vi "APC_9049_SAVE_loop.vi"(0 "DAQqueues":T1) -> ()   [LabVIEW 2020]
doc: "This example demonstrates the procedure required to apply different NI-DAQmx Custom Scales to each virtual channel in a task. A DAQmx Task Property Node (Functions >> NI Measurements >> DAQmx - Data Acquisition >> DAQmx Advanced Task Options) is used to obtain the task's virtual channels. A DAQmx Channel Property Node (Functions >> NI Measurements >> DAQmx - Data Acquisition) is then used to set the custom scale for each virtual channel in the task.\n\nThe \"DAQmx Create Scale\" VI creates a custom scale for each channel in the channel list. *Note, make sure your Minimum and Maximum channel parameters are consistent with the range the scale will create."
uses:
  controls/APC_DAQqueues.ctl
  controls/APC_SavingFile.ctl
  <vilib>/Platform/TimedLoop/XDataNode/timing_clust.ctl
  <vilib>/Platform/TimedLoop/XDataNode/nitl_modes.ctl
  <vilib>/Platform/TimedLoop/XDataNode/wakeup.ctl
  <vilib>/platform/TimedLoop/XDataNode/XDataNode.xnode
  <vilib>/Platform/TimedLoop/XDataNode/XDNodeRunTimeDep.lvlib
panel:
  in  "BufferingTImeLimit [s]":i32
  out "SignalList.CycAvg":string[](array[string])
  out "Cycles to measure":u16
  out "# elements in queue":i32
  out "Recorded cycles":i32
  out "TEST CODE":string
  out "No disk":bool=TRUE
  out "Full disk":bool
  out "size(s) 2":i32[](array[numeric])
  out "size(s)":i32[](array[numeric])
  out "Files and paths":T2
  out "error out 2":errorcluster
  out "error out":errorcluster
  in  "PostMortem":bool
  in  "AutoClearNote":bool
  out "ID":u32=6
  out "Test Notes":string
  out "FLUSH and SAVE BUFFER":bool
  out "REC BUFFER":bool
  in  "Stop File Saving Loop":bool
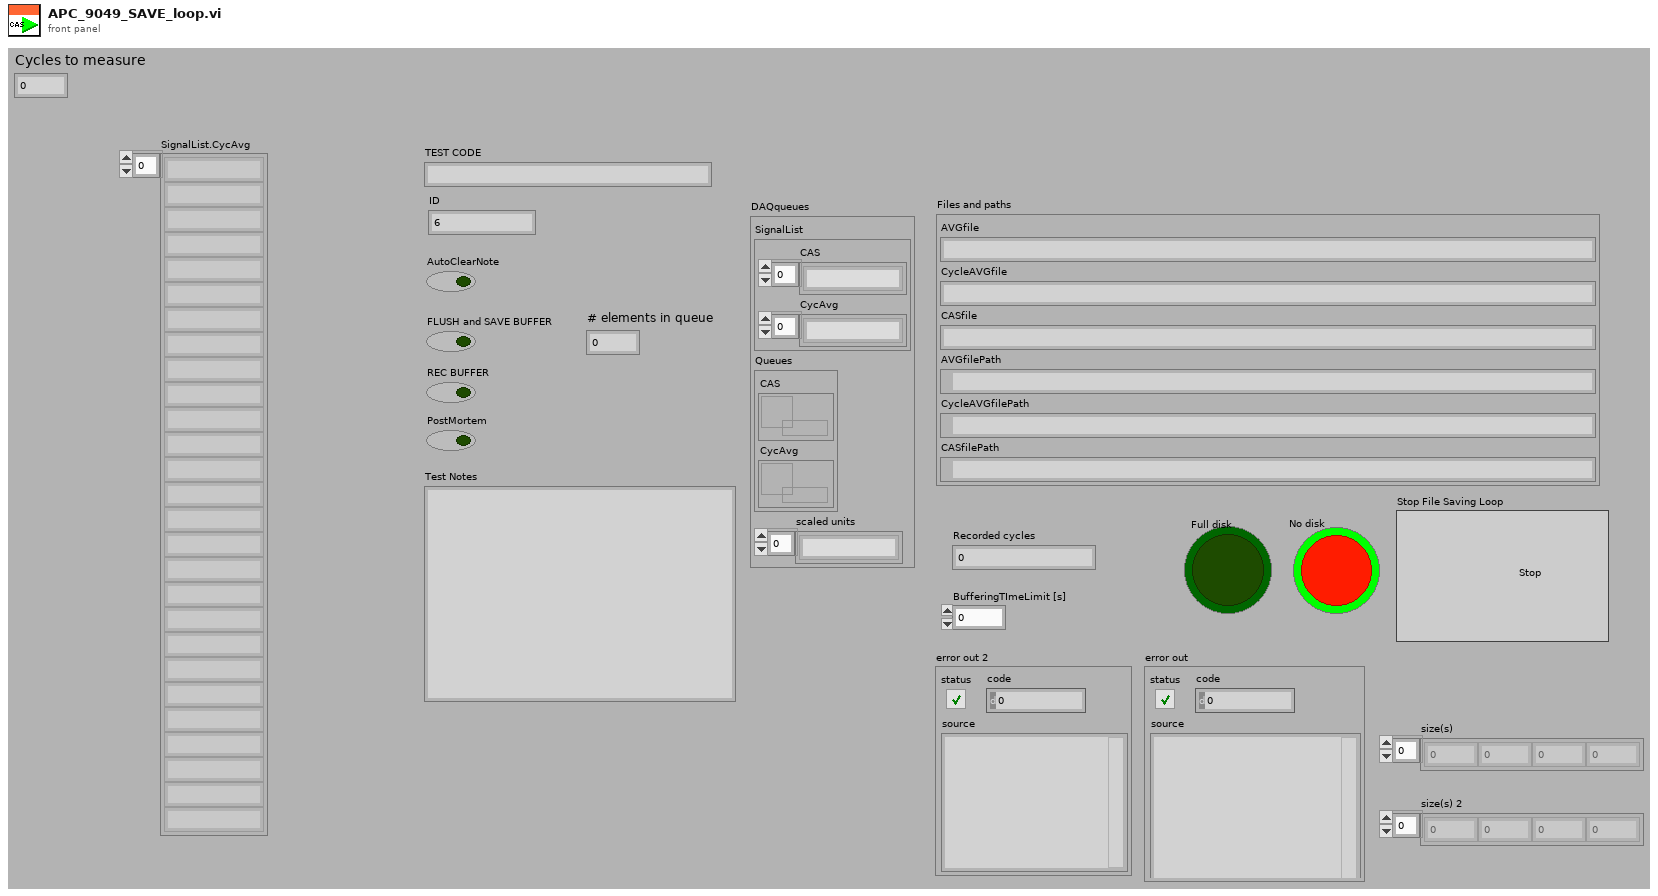
[diagram p1: front panel]
types:
  T1 = typedef "APC_DAQqueues.ctl" = cluster{"SignalList":cluster{"CAS":string[], "CycAvg":string[]}, "Queues":cluster{"CAS":refnum<queue>, "CycAvg":refnum<queue>}, "scaled units":string[]}
  T2 = cluster{"AVGfile":string, "CycleAVGfile":string, "CASfile":string, "AVGfilePath":path, "CycleAVGfilePath":path, "CASfilePath":path}
  T3 = enum16{"open", "open or create", "create or replace", "create", "open (read-only)"}
  T4 = typedef "XDNodeRunTimeDep.lvlib/timing_clust.ctl" = cluster{"Expected End [f-1]":u64, "Actual End [f-1]":u64, "Finished Late? [f-1]":bool, "Expected End [i-1]":u64, "Actual End [i-1]":u64, "Finished Late? [i-1]":bool, "Expected Start [i]":u64, "Actual Start [i]":u64, "Expected Start [f]":u64, "Actual Start [f]":u64, "Source Name":string, "Structure Name":string, "Period":i64, "Deadline":i64, "Offset":i64, "Start":i64, "Priority":i32, "Timeout":i32, "Mode":T5, "Wakeup Reason":T6, "Error":errorcluster, "Source Type":string, "Secondary Source Type":string, "Global End Time":u64, "Global Start Time":u64, "Frame Duration":u64, "Iteration Duration":u64, "Assigned CPU":i32, "I/O Scan Engine Mode":u32}
  T5 = typedef "XDNodeRunTimeDep.lvlib/nitl_modes.ctl" = enum32{"No Change", "Process missed periods, maintain original phase", "Discard missed periods, maintain original phase", "Process missed periods, ignore original phase", "Discard missed periods, ignore original phase"}
  T6 = typedef "XDNodeRunTimeDep.lvlib/wakeup.ctl" = enum32{"Normal", "Aborted", "Asynchronous wakeup", "Timing source error", "Timed loop error", "Timeout"}
  T7 = typedef "APC_SavingFile.ctl" = cluster{"TEST CODE":string, "ID":u32, "FLUSH and SAVE BUFFER":bool, "REC BUFFER":bool, "Test Notes":string, "Cycles":u16}
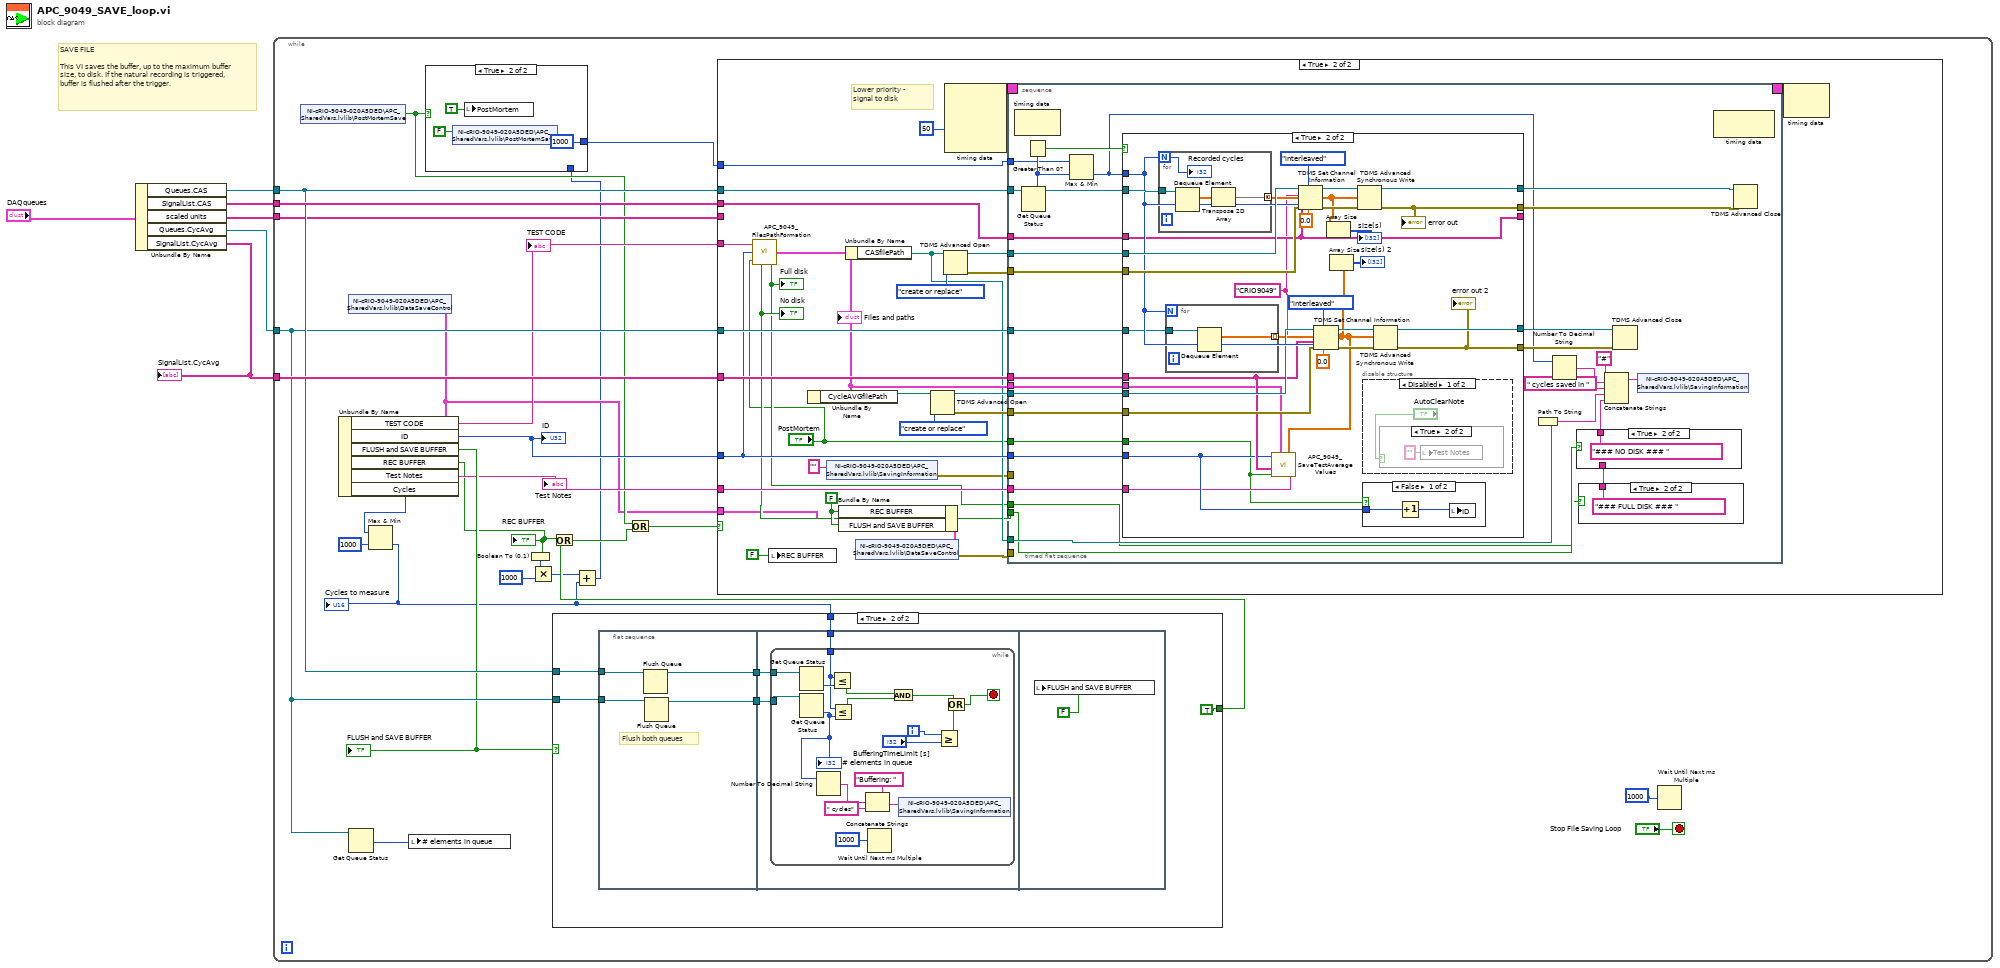
[diagram p0: block diagram]
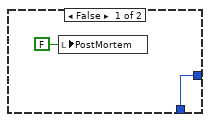
[diagram p2: hidden frame]
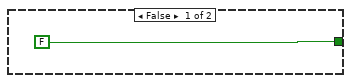
[diagram p3: hidden frame]
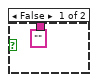
[diagram p5: hidden frame]
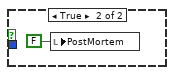
[diagram p10: hidden frame]
diagram:
  # "SAVE FILE\n\nThis VI saves the buffer, up to the maximum buffer size, to disk. If the natural recording is triggered, buffer is flushed after the trigger."
  n1 = Unbundle By Name("DAQqueues") -> ("Queues.CAS"=w6:refnum<queue>, "SignalList.CAS"=w5:string[], "scaled units"=w2:string[], "Queues.CycAvg"=w4:refnum<queue>, "SignalList.CycAvg"=w3:string[])
  "SignalList.CycAvg" <- w3
  n2 = while {
    tunnel: w6 -> [w28]
    tunnel: w5 -> [w32]
    tunnel: w4 -> [w25]
    tunnel: w3 -> [w30]
    tunnel: w2 -> [w26]
    stop <- "Stop File Saving Loop" stop-if-true
    n3 = shared-variable "NI-cRIO-9049-020A5DED\\APC_SharedVars.lvlib\\PostMortemSave"() -> (w12:bool)  [unwired: 1 in, 1 out]
    n4 = shared-variable "NI-cRIO-9049-020A5DED\\APC_SharedVars.lvlib\\DataSaveControl"() -> (w9:T7)  [unwired: 1 in, 1 out]
    n5 = Unbundle By Name(w9) -> ("TEST CODE"=w23:string, "ID"=w22:u32, "FLUSH and SAVE BUFFER"=w21:bool, "REC BUFFER"=w19:bool, "Test Notes"=w20:string, "Cycles"=w15:u16)
    "REC BUFFER" <- w19
    "FLUSH and SAVE BUFFER" <- w21
    "ID" <- w22
    "TEST CODE" <- w23
    "Test Notes" <- w20
    n6 = Get Queue Status(queue=w25) -> (# elements in queue=w24:i32)  [unwired: 2 in, 7 out]
    n7 = Max & Min(x=w15, y=u16 1000) -> (min(x,y)=w13:u16)  [unwired: 1 out]
    "Cycles to measure" <- w13
    n8 = local write "# elements in queue"(w24) -> ()
    n9 = Boolean To (0,1)(Boolean=w19) -> (0, 1=w18:i16)
    n10 = Multiply(x=w18, y=i16 1000) -> (x*y=w16:i16)
    n11 = case shown="True" w21 {
      tunnel: w28 -> [_ w44]
      tunnel: w25 -> [_ w43]
      tunnel: [FALSE TRUE] -> w27
      tunnel: w13 -> [_ w39]
      frame False {
      }
      frame True {
        n12 = flat-sequence {
          tunnel: w44 -> [w48]
          tunnel: w43 -> [w47]
          tunnel: [w46] -> w42
          tunnel: [w45] -> w41
          tunnel: w42 -> [w51]
          tunnel: w41 -> [w50]
          tunnel: w39 -> [w49]
          frame #0 {
            # "Flush both queues"
            n13 = Flush Queue(queue=w48) -> (queue out=w46:refnum<queue>)  [unwired: 1 in, 2 out]
            n14 = Flush Queue(queue=w47) -> (queue out=w45:refnum<queue>)  [unwired: 1 in, 2 out]
          }
          frame #1 {
            n15 = while {
              tunnel: w51 -> [w68]
              tunnel: w50 -> [w67]
              tunnel: w49 -> [w57]
              i -> [w53]
              stop <- w55 stop-if-true
              n16 = Get Queue Status(queue=w68) -> (# elements in queue=w66:i32)  [unwired: 2 in, 7 out]
              n17 = Get Queue Status(queue=w67) -> (# elements in queue=w60:i32)  [unwired: 2 in, 7 out]
              "# elements in queue" <- w60
              n18 = Number To Decimal String(number=w60) -> (decimal integer string=w62:string)  [unwired: 1 in]
              n19 = Less Or Equal?(x=w57, y=w66) -> (x <= y?=w65:bool)
              n20 = Less Or Equal?(x=w57, y=w60) -> (x <= y?=w64:bool)
              n21 = Concatenate Strings("Buffering: " ("string"), w62, " cycles" ("string")) -> (w61:string)
              n22 = Wait Until Next ms Multiple(millisecond multiple=u32 1000) -> ()  [unwired: 1 out]
              n23 = And(x=w65, y=w64) -> (x .and. y?=w56:bool)
              n24 = shared-variable "NI-cRIO-9049-020A5DED\\APC_SharedVars.lvlib\\SavingInformation"(w61) -> ()  [unwired: 1 in, 1 out]
              n25 = Greater Or Equal?(x=w53, y="BufferingTImeLimit [s]") -> (x >= y?=w54:bool)
              n26 = Or(x=w56, y=w54) -> (x .or. y?=w55:bool)
            }
          }
          frame #2 {
            n27 = local write "FLUSH and SAVE BUFFER"(FALSE) -> ()
          }
        }
      }
    }
    n28 = Or(x=w19, y=w27) -> (x .or. y?=w11:bool)
    n29 = Add(x=w16, y=w13) -> (x+y=w8:u16)
    n30 = case shown="True" w12 {
      tunnel: w8 -> [w33 _]
      tunnel: [w33 u16 1000] -> w7
      frame False {
        n31 = local write "PostMortem"(FALSE ("PostMortem")) -> ()
      }
      frame True {
        n32 = shared-variable "NI-cRIO-9049-020A5DED\\APC_SharedVars.lvlib\\PostMortemSave"(FALSE ("PostMortemSave")) -> ()  [unwired: 1 in, 1 out]
        n33 = local write "PostMortem"(TRUE ("PostMortem")) -> ()
      }
    }
    n34 = Or(x=w12, y=w11) -> (x .or. y?=w10:bool)
    n35 = case shown="True" w10 {
      tunnel: w28 -> [_ w96]
      tunnel: w32 -> [_ w72]
      tunnel: w25 -> [_ w93]
      tunnel: w30 -> [_ w92]
      tunnel: w26 -> [_ _]
      tunnel: w22 -> [_ w84]
      tunnel: w23 -> [_ w83]
      tunnel: w20 -> [_ w82]
      tunnel: w7 -> [_ w75]
      tunnel: w9 -> [_ w71]
      frame False {
      }
      frame True {
        w79 = FALSE ("REC BUFFER")
        # "Lower priority - signal to disk"
        n36 = call "APC_9049_FilesPathFormation.vi"("PostMortem"="PostMortem", "ID"=w84, "TEST CODE"=w83) -> ("Full disk"=w73:bool, "No disk"=w74:bool, "Files and paths"=w85:T2)
        "Files and paths" <- w85
        "Full disk" <- w73
        "No disk" <- w74
        n37 = local write "REC BUFFER"(FALSE ("SAVE")) -> ()
        n38 = Unbundle By Name(w85) -> ("CycleAVGfilePath"=w86:path)
        n39 = shared-variable "NI-cRIO-9049-020A5DED\\APC_SharedVars.lvlib\\SavingInformation"("" ("SavingInformation")) -> (error out=w77:errorcluster)  [unwired: 1 in]
        n40 = Bundle By Name(cluster=w71, "REC BUFFER"=w79, "FLUSH and SAVE BUFFER"=w79) -> (w80:T7)
        n41 = Unbundle By Name(w85) -> ("CASfilePath"=w81:path)
        n42 = shared-variable "NI-cRIO-9049-020A5DED\\APC_SharedVars.lvlib\\DataSaveControl"(w80) -> (error out=w76:errorcluster)  [unwired: 1 in]
        n43 = TDMS Advanced Open(10:T3."create or replace" ("operation (0:open)"), 11:w86) -> (0:w90:errorcluster, 3:w91:refnum<k34>)  [unwired: 3 in, 1 out]
        n44 = TDMS Advanced Open(10:T3."create or replace" ("operation (0:open)"), 11:w81) -> (0:w94:errorcluster, 3:w95:refnum<k34>)  [unwired: 3 in, 1 out]
        n45 = node-c288(50 ("Priority")) -> (w99:T4)  [unwired: 3 in]
        n46 = timed-sequence {
          timing: w99 -> [_]
          timing-out: [_] -> w98
          tunnel: w96 -> [w117]
          tunnel: w72 -> [w116]
          tunnel: w95 -> [w115]
          tunnel: w94 -> [w114]
          tunnel: w93 -> [w113]
          tunnel: w92 -> [w112]
          tunnel: w91 -> [w111]
          tunnel: w90 -> [w110]
          tunnel: w84 -> [w109]
          tunnel: w85 -> [w108]
          tunnel: w82 -> [w107]
          tunnel: w81 -> [w106]
          tunnel: w77 -> [w105]
          tunnel: w76 -> [w104]
          tunnel: w75 -> [w103]
          tunnel: w74 -> [w102]
          tunnel: w73 -> [w101]
          tunnel: "PostMortem" -> [w100]
          n47 = timed-flat-sequence {
            tunnel: w117 -> [w148]
            tunnel: w116 -> [w147]
            tunnel: w115 -> [w146]
            tunnel: w114 -> [w145]
            tunnel: w113 -> [w144]
            tunnel: w112 -> [w143]
            tunnel: w111 -> [w140]
            tunnel: w110 -> [w139]
            tunnel: w109 -> [w136]
            tunnel: w108 -> [w135]
            tunnel: w107 -> [w132]
            tunnel: w106 -> [w130]
            tunnel: w105 -> [_]
            tunnel: w104 -> [_]
            tunnel: w103 -> [w123]
            tunnel: w102 -> [w120]
            tunnel: w101 -> [w119]
            tunnel: w100 -> [w118]
            n48 = node-c288() -> ()  [unwired: 1 in, 1 out]
            n49 = Get Queue Status(queue=w148) -> (queue out=w142:refnum<queue>, # elements in queue=w125:i32)  [unwired: 2 in, 6 out]
            n50 = Greater Than 0?(x=w125) -> (x > 0?=w141:bool)
            n51 = Max & Min(x=w123, y=w125) -> (min(x,y)=w124:i32)  [unwired: 1 out]
            n52 = case shown="True" w141 {
              tunnel: w142 -> [_ w187]
              tunnel: w124 -> [_ w176]
              tunnel: w147 -> [w153 w161]
              tunnel: [w157 w183] -> w133
              tunnel: [w156 w182] -> w134
              tunnel: w146 -> [w157 w181]
              tunnel: w145 -> [w156 w180]
              tunnel: w144 -> [_ w175]
              tunnel: w143 -> [_ w170]
              tunnel: w140 -> [w155 w174]
              tunnel: w139 -> [w154 w173]
              tunnel: [w155 w172] -> w138
              tunnel: [w154 w171] -> w137
              tunnel: w136 -> [_ w168]
              tunnel: w135 -> [_ w169]
              tunnel: [w153 w161] -> _
              tunnel: w132 -> [_ w159]
              tunnel: w118 -> [_ w158]
              frame False {
              }
              frame True {
                w160 = "CRIO9049" ("group name (Untitled)")
                n53 = for {
                  N: w176 -> [w195]
                  tunnel: w187 -> [w198]
                  tunnel: [w196] -> w165 mode=concatenating
                  n54 = Dequeue Element(queue=w198) -> (element=w197:dbl[][])  [unwired: 2 in, 3 out]
                  n55 = Transpose 2D Array(2D array=w197) -> (transposed array=w196:dbl[][])
                  "Recorded cycles" <- w195
                }
                n56 = for {
                  N: w176 -> [_]
                  tunnel: w175 -> [w194]
                  tunnel: [w193] -> w162 mode=indexing
                  n57 = Dequeue Element(queue=w194) -> (element=w193:dbl[])  [unwired: 2 in, 3 out]
                }
                n58 = call "APC_9049_SaveTestAverageValues.vi"("ID"=w168, "Data Array"=w162, "Signals"=w170, "PostMortem"=w158, "Files and paths"=w169, "Test Notes"=w159) -> ()  [unwired: 1 in]
                n59 = TDMS Set Channel Information(4:w176, 6:0.0 ("data type"), 7:enum16{"non-interleaved", "interleaved"}."interleaved" ("data layout (0:non-interleaved)"), 8:w180, 9:w161, 10:w160, 11:w181) -> (0:w184:errorcluster, 3:w185:refnum<k34>)
                n60 = TDMS Set Channel Information(4:w176, 6:0.0 ("data type"), 7:enum16{"non-interleaved", "interleaved"}."interleaved" ("data layout (0:non-interleaved)"), 8:w173, 9:w170, 10:w160, 11:w174) -> (0:w177:errorcluster, 3:w178:refnum<k34>)
                n61 = Array Size(array=w165) -> (size(s)=→"size(s)":i32[])
                n62 = Array Size(array=w162) -> (size(s)=→"size(s) 2":i32[])
                n63 = TDMS Advanced Synchronous Write(8:w184, 10:w165, 11:w185) -> (0:w182:errorcluster, 3:w183:refnum<k34>)
                "error out" <- w182
                n64 = disable-structure shown="Disabled" {
                  frame Disabled {
                    n65 = case shown="True" "AutoClearNote" {
                      frame False {
                      }
                      frame True {
                        n66 = local write "Test Notes"("" ("Test Notes")) -> ()
                      }
                    }
                  }
                  frame Enabled {
                  }
                }
                n67 = case shown="False" w158 {
                  tunnel: w168 -> [w191 _]
                  frame False {
                    n68 = Increment(x=w191) -> (x+1=w190:u32)
                    n69 = local write "ID"(w190) -> ()
                  }
                  frame True {
                    n70 = local write "PostMortem"(FALSE ("PostMortem")) -> ()
                  }
                }
                n71 = TDMS Advanced Synchronous Write(8:w177, 10:w162, 11:w178) -> (0:w171:errorcluster, 3:w172:refnum<k34>)
                "error out 2" <- w171
              }
            }
            n72 = Path To String(path=w130) -> (string=w131:string)
            n73 = Number To Decimal String(number=w124) -> (decimal integer string=w129:string)  [unwired: 1 in]
            n74 = case shown="True" w119 {
              tunnel: ["" ("string") "### FULL DISK ### " ("string")] -> w121
              frame False {
              }
              frame True {
              }
            }
            n75 = case shown="True" w120 {
              tunnel: [w151 "### NO DISK ### " ("string")] -> w122
              tunnel: w121 -> [w151 _]
              frame False {
              }
              frame True {
              }
            }
            n76 = Concatenate Strings("#" ("string"), w129, " cycles saved in " ("string"), w131, w122) -> (w127:string)
            n77 = TDMS Advanced Close(8:w137, 11:w138) -> ()  [unwired: 2 in, 2 out]
            n78 = shared-variable "NI-cRIO-9049-020A5DED\\APC_SharedVars.lvlib\\SavingInformation"(w127) -> ()  [unwired: 1 in, 1 out]
            n79 = node-c288() -> ()  [unwired: 1 in, 1 out]
            n80 = TDMS Advanced Close(8:w134, 11:w133) -> ()  [unwired: 2 in, 2 out]
          }
        }
        n81 = node-c288(w98) -> ()  [unwired: 1 out]
      }
    }
    n82 = Wait Until Next ms Multiple(millisecond multiple=u32 1000) -> ()  [unwired: 1 out]
  }
